vi "Pre Launch Init.vi"(11 "Nested in":refnum<class "Stage Controller StepMotor.lvclass">) -> (0 "error out":errorcluster, 3 "Nested out":refnum<class "Stage Controller StepMotor.lvclass">)   [LabVIEW 2020, in "Stage.lvlib" / "Stage Controller StepMotor.lvlib" / "Stage Controller StepMotor.lvclass"]
doc: "(<B>Filename</B>: Actor Framework.lvlib:Actor.lvclass:Pre Launch Init.vi)\n\nDefines behavior that occurs after the Launch Nested Actor method is invoked but before the actor's Actor Core method begins running.\n\nBy default, this method does nothing. A descendant class may override it to define behavior."
uses:
  Stage Controller StepMotor.lvclass
  Stage Controller StepMotor.lvclass/Stage Controller StepMotor.ctl
  <vilib>/ActorFramework/Actor/Actor.lvclass
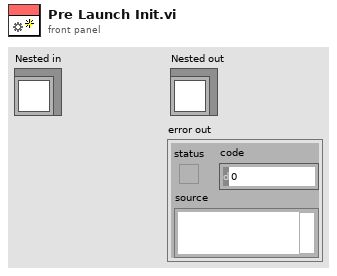
[diagram p1: front panel]
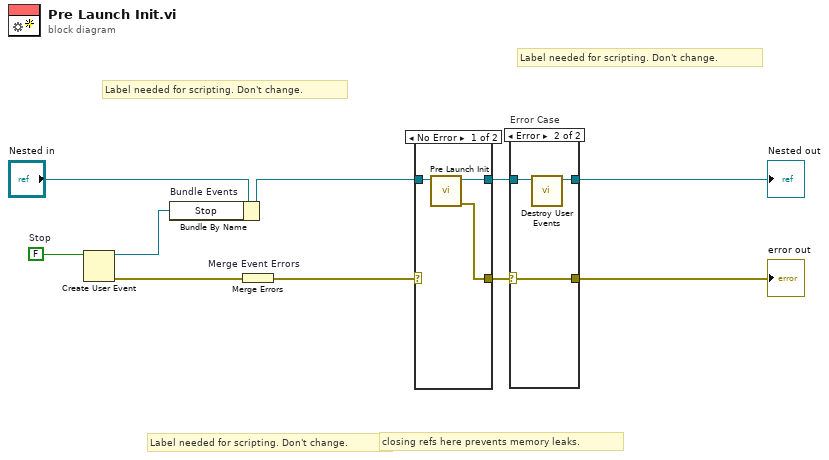
[diagram p0: block diagram]
diagram:
  w9 = FALSE  # Stop
  # "Label needed for scripting. Don't change."
  # "Label needed for scripting. Don't change."
  # "Label needed for scripting. Don't change."
  # "closing refs here prevents memory leaks."
  n1 = Create User Event(user event datatype=w9) -> (user event=w6:refnum<user-event>, error out=w8:errorcluster)  [unwired: 1 in]
  n2 = Bundle By Name "Bundle Events"(cluster="Nested in", "Stop"=w6) -> (w3:refnum<class "Stage Controller StepMotor.lvclass">)
  n3 = Merge Errors "Merge Event Errors"(w8) -> (w2:errorcluster)
  n4 = case shown="No Error" w2 {
    selector: w2 -> [_ w15]
    tunnel: [w13 w14] -> w4
    tunnel: w3 -> [w12 w14]
    tunnel: [w11 w15] -> w1
    frame No Error {
      n5 = call-parent "Pre Launch Init.vi"("Actor in"=w12) -> ("error out"=w11:errorcluster, "Actor out"=w13:refnum<class "Stage Controller StepMotor.lvclass">)  [unwired: 9 in]
    }
    frame Error {
    }
  }
  n6 = case "Error Case" shown="Error" w1 {
    selector: w1 -> [w16 w20]
    tunnel: w4 -> [w17 w19]
    tunnel: [w17 w18] -> w7
    tunnel: [w16 w20] -> w5
    frame No Error {
    }
    frame Error {
      n7 = call "Destroy User Events.vi"("UI Template in"=w19) -> ("UI Template out"=w18:refnum<class "Stage Controller StepMotor.lvclass">)  [unwired: 10 in]
    }
  }
  "error out" <- w5
  "Nested out" <- w7
